vi "Daq2.vi"() -> ()   [LabVIEW 2020]
uses:
  <extravilib>/ChannelInstances/Tag-bool/Read With Abort.vi
  <extravilib>/ChannelInstances/Tag-bool/Write With Abort.vi
  <extravilib>/ChannelInstances/Tag-bool/Instantiate.vi
  <extravilib>/ChannelInstances/Tag-bool/EndpointRead.vi
  <extravilib>/ChannelInstances/Tag-bool/Endpoint.vi
  <extravilib>/ChannelInstances/Tag-bool.lvlib
panel:
  in  "?":bool
  out "RPM":dbl
  out "RPM":dbl(knob) scale=1790.0..1800.0
  in  "Number of teeth in gear":dbl
  out "Signal Frequency (Hz)":dbl format="%#_13g"
  in  "Sample rate":dbl=1000.0
  in  "Number of Samples":i32=5
  in  "Voltage Threshold":dbl
  out "dt":dbl
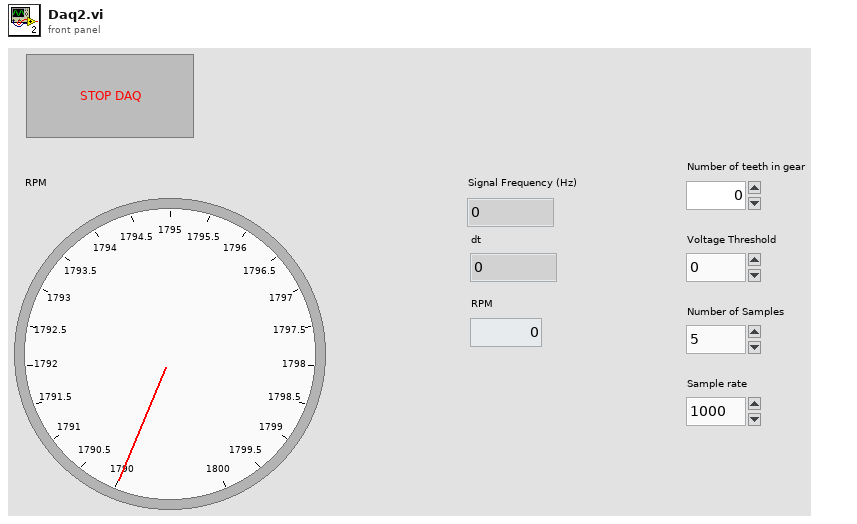
[diagram p1: front panel]
types:
  T1 = typedef "Tag-bool.lvlib/))Channel.ctl" = refnum<queue>
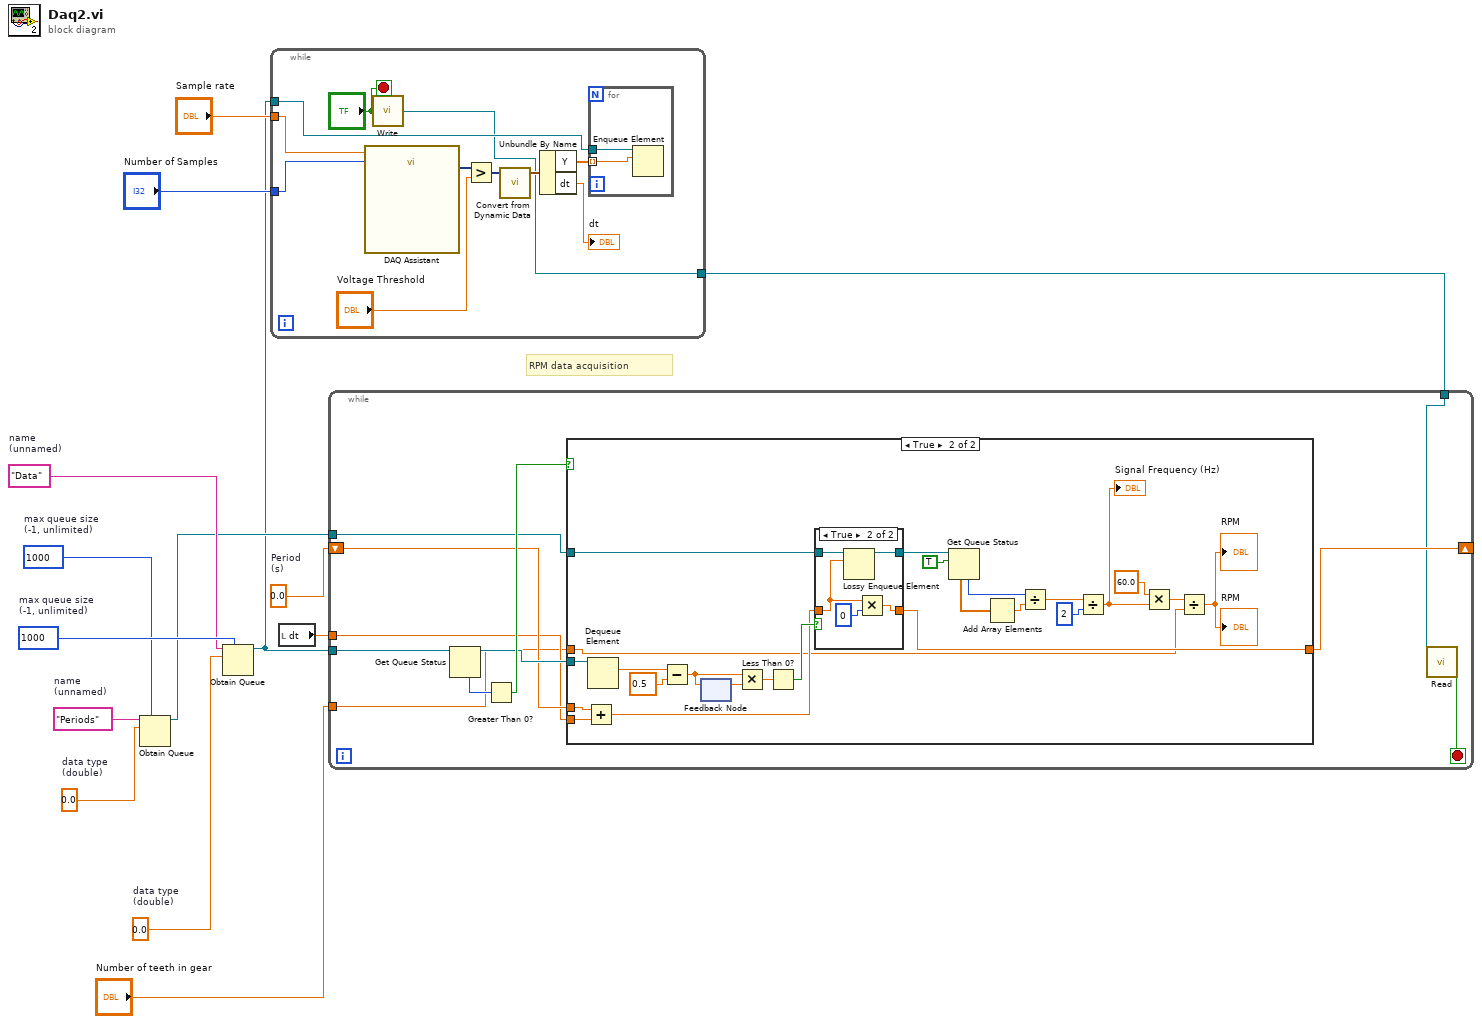
[diagram p0: block diagram]
diagram:
  w4 = 0.0  # Period (s)
  w9 = 0.0  # data type (double)
  w10 = "Periods"  # name (unnamed)
  w11 = 1000  # max queue size (-1, unlimited)
  w12 = 0.0  # data type (double)
  w13 = "Data"  # name (unnamed)
  w14 = 1000  # max queue size (-1, unlimited)
  # "RPM data acquisition"
  n1 = Obtain Queue(max queue size (-1, unlimited)=w11, name (unnamed)=w10, element data type=w9) -> (queue out=w6:refnum<queue>)  [unwired: 2 in, 2 out]
  n2 = Obtain Queue(max queue size (-1, unlimited)=w14, name (unnamed)=w13, element data type=w12) -> (queue out=w5:refnum<queue>)  [unwired: 2 in, 2 out]
  n3 = while {
    tunnel: w5 -> [w23]
    tunnel: "Sample rate" -> [w19]
    tunnel: "Number of Samples" -> [w18]
    tunnel: [w15] -> w1
    stop <- "?" stop-if-true
    n4 = call "DAQ Assistant"("rate"=w19, "number of samples"=w18) -> ("data"=w17:dynamicdata)  [unwired: 14 in, 3 out]
    n5 = call <extravilib>:"Write.vi"("element"="?") -> ("channel"=w15:T1)  [unwired: 1 out]
    n6 = Greater?(x=w17, y="Voltage Threshold") -> (0:w21:dynamicdata)
    n7 = call "Convert from Dynamic Data"("Dynamic Data Type"=w21) -> ("Waveform"=w25:waveform(dbl))  [unwired: 3 in]
    n8 = Unbundle By Name(w25) -> ("Y"=w24:dbl[], "dt"=→"dt":dbl)
    n9 = for {
      tunnel: w24 -> [w27] mode=indexing
      tunnel: w23 -> [w26]
      n10 = Enqueue Element(queue=w26, element=w27) -> ()  [unwired: 2 in, 3 out]
    }
  }
  n11 = local read "dt"() -> (w3:dbl)
  n12 = while {
    tunnel: w5 -> [w37]
    tunnel: w6 -> [w34]
    shift-right: [w31] -> _
    shift-left: w4 -> [w33]
    tunnel: w3 -> [w32]
    tunnel: "Number of teeth in gear" -> [w30]
    tunnel: w1 -> [w28]
    stop <- w29 stop-if-true
    n13 = Get Queue Status(queue=w37) -> (queue out=w35:refnum<queue>, # elements in queue=w38:i32)  [unwired: 2 in, 6 out]
    n14 = Greater Than 0?(x=w38) -> (x > 0?=w36:bool)
    n15 = case shown="True" w36 {
      tunnel: w35 -> [_ w63]
      tunnel: w34 -> [_ w57]
      tunnel: w33 -> [w39 w47]
      tunnel: w32 -> [_ w46]
      tunnel: [w39 w49] -> w31
      tunnel: w30 -> [_ w41]
      frame False {
      }
      frame True {
        n16 = Add(x=w47, y=w46) -> (x+y=w45:dbl)
        n17 = Dequeue Element(queue=w63) -> (element=w62:dbl)  [unwired: 2 in, 3 out]
        n18 = Subtract(x=w62, y=0.5) -> (x-y=w60:dbl)
        n19 = feedback-in #1(w60) -> ()
        n20 = feedback #1() -> (w59:dbl)  [unwired: 1 in]
        n21 = Multiply(x=w60, y=w59) -> (x*y=w58:dbl)
        n22 = Less Than 0?(x=w58) -> (x < 0?=w48:bool)
        n23 = case shown="True" w48 {
          tunnel: w57 -> [w65 w69]
          tunnel: [w65 w68] -> w55
          tunnel: [w64 w67] -> w49
          tunnel: w45 -> [w64 w66]
          frame False {
          }
          frame True {
            n24 = Lossy Enqueue Element(queue=w69, element=w66) -> (queue out=w68:refnum<queue>)  [unwired: 1 in, 3 out]
            n25 = Multiply(x=w66, y=0) -> (x*y=w67:dbl)
          }
        }
        n26 = Get Queue Status(queue=w55, return elements? (F)=TRUE) -> (# elements in queue=w50:i32, elements=w54:dbl[])  [unwired: 1 in, 6 out]
        n27 = Add Array Elements(numeric array=w54) -> (sum=w51:dbl)
        n28 = Divide(x=w50, y=w51) -> (x/y=w52:dbl)
        n29 = Divide(x=w52, y=2) -> (x/y=w43:dbl)
        "Signal Frequency (Hz)" <- w43
        n30 = Multiply(x=60.0, y=w43) -> (x*y=w42:dbl)
        n31 = Divide(x=w42, y=w41) -> (x/y=→"RPM" →"RPM":dbl)
      }
    }
    n32 = call <extravilib>:"Read.vi"("channel"=w28) -> ("element"=w29:bool)  [unwired: 1 in, 1 out]
  }
